vi "Extract View from 2D Array.vi"(9 "Column":i32, 10 "Row":i32, 11 "Board Array":i32[][](array[numeric])=[[1, 11, 10, 111, 101], [2, 22, 20, 222, 102], [3, 33, 30, 333, 103], [4, 44, 40, 444, 104], [5, 55, 50, 555, 105]]) -> (2 "View Out":i32[](array[numeric]), 3 "Directions Out":T1[](array[typedef])=[enum."NW", enum."N", enum."NE", enum."E", enum."SE", enum."S", enum."S", enum."SW", enum."W"])   [LabVIEW 2017, in "AntFarm_MB.lvclass"]
uses:
  AntFarm_MB.lvclass
  Type Defs/Direction Enum.ctl
  Type Defs/SB Type Defs.lvlib
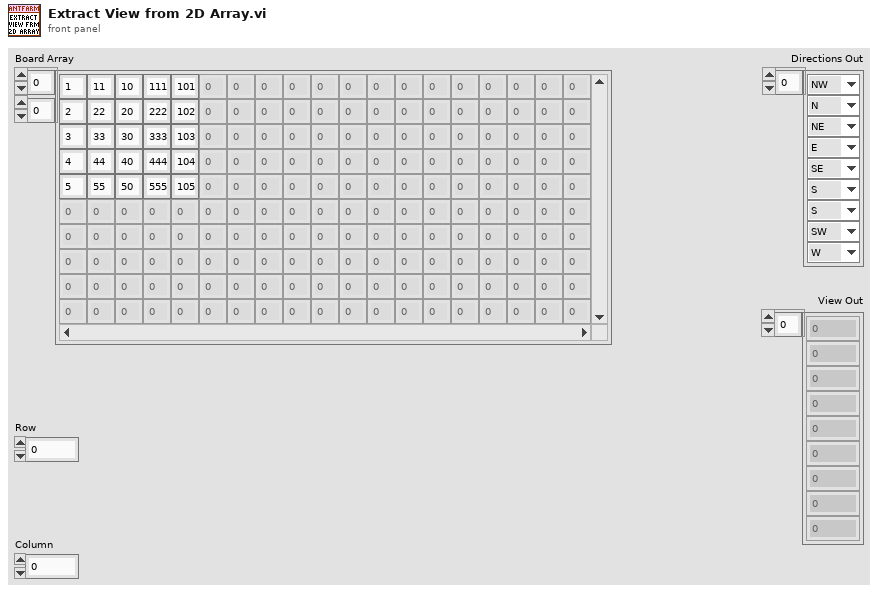
[diagram p1: front panel]
types:
  T1 = typedef "SB Type Defs.lvlib/Direction Enum.ctl" = enum16{"NW", "N", "NE", "E", "SE", "S", "SW", "W"}
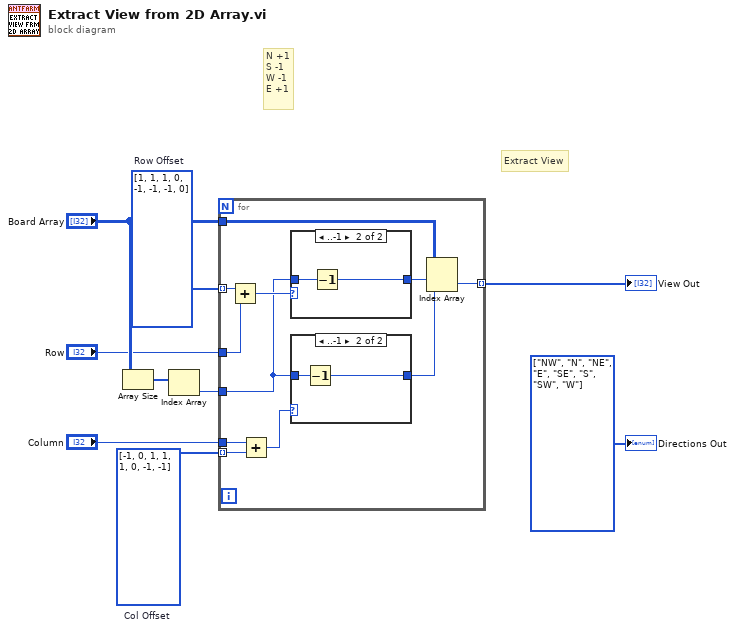
[diagram p0: block diagram]
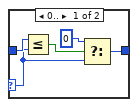
[diagram p2: hidden frame]
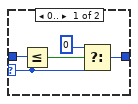
[diagram p3: hidden frame]
diagram:
  w2 = i32[] [1, 1, 1, 0, -1, -1, -1, 0]  # Row Offset
  w1 = i32[] [-1, 0, 1, 1, 1, 0, -1, -1]  # Col Offset
  w5 = T1[] [enum."NW", enum."N", enum."NE", enum."E", enum."SE", enum."S", enum."SW", enum."W"] items=["NW", "N", "NE", "E", "SE", "S", "SW", "W"] ("Directions Out")
  # "N +1\nS -1\nW -1\nE +1"
  # "Extract View"
  n1 = Array Size(array="Board Array") -> (size(s)=w4:i32[])
  n2 = Index Array(array=w4) -> (element=w3:i32)  [unwired: 1 in]
  n3 = for {
    tunnel: "Board Array" -> [w13]
    tunnel: w3 -> [w14]
    tunnel: w2 -> [w19] mode=indexing
    tunnel: w1 -> [w16] mode=indexing
    tunnel: "Row" -> [w20]
    tunnel: "Column" -> [w17]
    tunnel: [w10] -> w6 mode=indexing
    n4 = Add(x=w19, y=w20) -> (x+y=w18:i32)
    n5 = Add(x=w17, y=w16) -> (x+y=w15:i32)
    n6 = case shown="..-1" w18 {
      selector: w18 -> [w30 _]
      tunnel: w14 -> [w29 w34]
      tunnel: [w28 w33] -> w12
      frame 0.. {
        n7 = Less Or Equal?(x=w29, y=w30) -> (x <= y?=w31:bool)
        n8 = Select(t=0, s=w31, f=w30) -> (s? t:f=w28:i32)
      }
      frame ..-1 {
        n9 = Decrement(x=w34) -> (x-1=w33:i32)
      }
    }
    n10 = case shown="..-1" w15 {
      selector: w15 -> [w23 _]
      tunnel: w14 -> [w25 w27]
      tunnel: [w22 w26] -> w11
      frame 0.. {
        n11 = Less Or Equal?(x=w25, y=w23) -> (x <= y?=w24:bool)
        n12 = Select(t=0, s=w24, f=w23) -> (s? t:f=w22:i32)
      }
      frame ..-1 {
        n13 = Decrement(x=w27) -> (x-1=w26:i32)
      }
    }
    n14 = Index Array(array=w13, index (row)=w12, index (col)=w11) -> (element=w10:i32)
  }
  "View Out" <- w6
  "Directions Out" <- w5
